vi "Pass If Specific Error.vi"(6 "Error Codes":i32[](array[numeric]), 7 "Description":string, 8 "error in (no error)":errorcluster, 10 "Assert error":errorcluster, 11 "LUnit Test Case In":refnum<class "LUnit Test Case.lvclass">) -> (0 "error out":errorcluster, 3 "LUnit Test Case Out":refnum<class "LUnit Test Case.lvclass">)   [LabVIEW 2020, in "Advanced Assertions.lvlib"]
doc: "Generates a pass result for the calling test method if the inputs contains an error with status \"True\". Using the Error Codes input it is possible to select which specific error codes to test for. A description may be provided to the result."
uses:
  Advanced Assertions.lvlib
  LUnit Test Case.lvclass
  LUnit Test Case.lvclass/LUnit Test Case.ctl
  d0e67a5c-31db-4060-a993-98defbf94426.vi
  Core/LUnit Test Case/Private/Append Fail Result.vi
  Core/LUnit Test Case/Private/Append Pass Result.vi
  Core/LUnit Test Case/Private/Run In UI.vi
  <vilib>/Utility/error.llb/Clear Errors.vi
  <vilib>/Comparison/Equal/Equal Functor/Equal Functor.lvclass
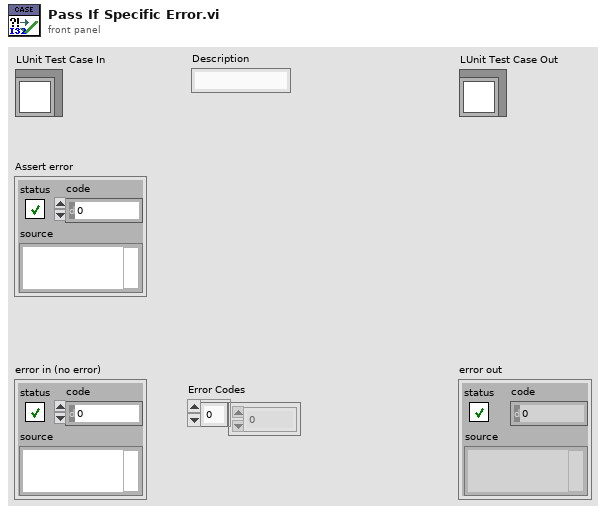
[diagram p1: front panel]
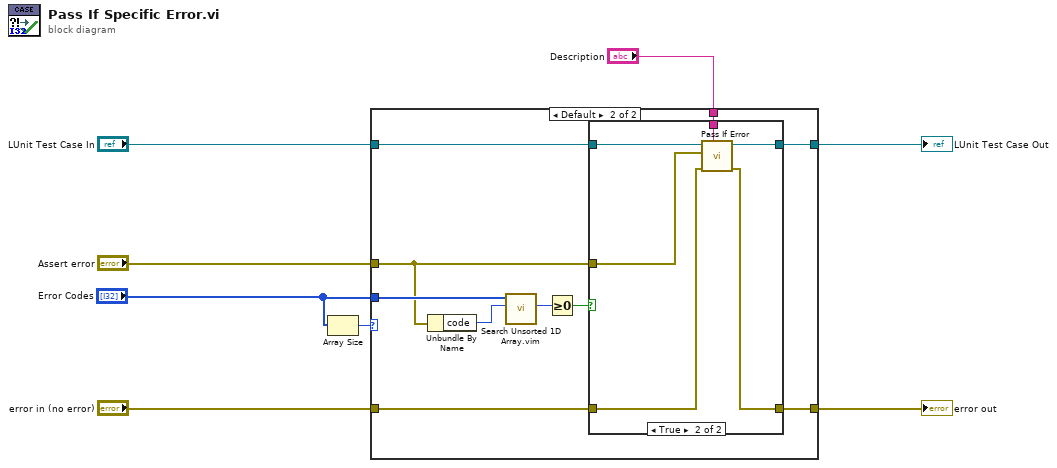
[diagram p0: block diagram]
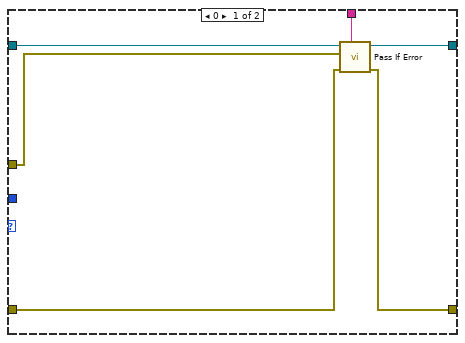
[diagram p2: hidden frame]
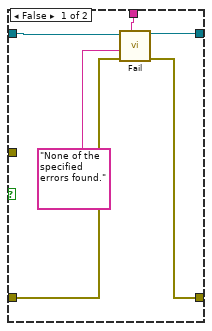
[diagram p3: hidden frame]
diagram:
  n1 = Array Size(array="Error Codes") -> (size(s)=w2:i32)
  n2 = case shown="Default" w2 {
    tunnel: "LUnit Test Case In" -> [w10 w24]
    tunnel: [w14 w23] -> w1
    tunnel: [w13 w22] -> w6
    tunnel: "Assert error" -> [w9 w16]
    tunnel: "Description" -> [w12 w21]
    tunnel: "error in (no error)" -> [w11 w20]
    tunnel: "Error Codes" -> [_ w19]
    frame 0 {
      n3 = call "Pass If Error.vi"("Description"=w12, "error in (no error)"=w11, "Assert error"=w9, "LUnit Test Case In"=w10) -> ("error out"=w13:errorcluster, "LUnit Test Case Out"=w14:refnum<class "LUnit Test Case.lvclass">)  [unwired: 6 in]
    }
    frame Default {
      n4 = Unbundle By Name(w16) -> ("code"=w15:i32)
      n5 = call "Search Unsorted 1D Array.vim"("element"=w15, "unsorted 1D array"=w19) -> ("index of element"=w18:i32)  [unwired: 9 in]
      n6 = Greater Or Equal To 0?(x=w18) -> (x >= 0?=w17:bool)
      n7 = case shown="True" w17 {
        tunnel: w24 -> [w28 w36]
        tunnel: [w27 w35] -> w23
        tunnel: [w29 w34] -> w22
        tunnel: w21 -> [w26 w33]
        tunnel: w20 -> [w30 w32]
        tunnel: w16 -> [_ w31]
        frame False {
          n8 = call "Fail.vi"("Description"=w26, "error in (no error)"=w30, "Message"="None of the specified errors found.", "LUnit Test Case In"=w28) -> ("error out"=w29:errorcluster, "LUnit Test Case Out"=w27:refnum<class "LUnit Test Case.lvclass">)  [unwired: 6 in]
        }
        frame True {
          n9 = call "Pass If Error.vi"("Description"=w33, "error in (no error)"=w32, "Assert error"=w31, "LUnit Test Case In"=w36) -> ("error out"=w34:errorcluster, "LUnit Test Case Out"=w35:refnum<class "LUnit Test Case.lvclass">)  [unwired: 6 in]
        }
      }
    }
  }
  "error out" <- w6
  "LUnit Test Case Out" <- w1
